vi "Update Controller State.vi"(8 "error in (no error)":errorcluster, 11 "ATM Controller in":refnum<class "ATM Controller.lvclass">) -> (0 "error out":errorcluster, 3 "ATM Controller out":refnum<class "ATM Controller.lvclass">)   [LabVIEW 2019, in "ATM Controller.lvlib" / "ATM Controller.lvclass"]
uses:
  ATM Controller.lvclass
  C:/Program Files (x86)/National Instruments/LabVIEW 2019/vi.lib/ActorFramework/Actor/Actor.lvclass
  <vilib>/ActorFramework/Actor/Actor.lvclass/Actor.ctl
  <vilib>/ActorFramework/Message Enqueuer/Message Enqueuer.lvclass/Message Enqueuer.ctl
  ATM Controller.lvclass/ATM Controller.ctl
  Sim Display Console Actor/ATM Controller/Transaction -Enum.ctl
  Sim Display Console Actor/ATM Controller/Message Name.ctl
  ATM Controller Messages/Set Message Msg/Set Message Msg.lvclass/Set Message Msg.ctl
  Sim User Console Actor/Sim User Console Actor Messages/Enable Transactions Msg/Enable Transactions Msg.lvclass/Enable Transactions Msg.ctl
  Sim User Console Actor/Sim User Console Actor Messages/Enable Keypad Msg/Enable Keypad Msg.lvclass/Enable Keypad Msg.ctl
  Sim User Console Actor/Sim User Console Actor Messages/Enable Card reader Msg/Enable Card reader Msg.lvclass/Enable Card reader Msg.ctl
  Sim Sensor Interface Actor/Sim Sensor Interface Actor Messages/Enable All Controls Msg/Enable All Controls Msg.lvclass/Enable All Controls Msg.ctl
  Sim Display Console Actor/Sim Display Console Actor Messages/Write Transaction Msg/Write Transaction Msg.lvclass/Write Transaction Msg.ctl
  Sim Display Console Actor/Sim Display Console Actor Messages/Write Card Read Msg/Write Card Read Msg.lvclass/Write Card Read Msg.ctl
  State -Enum.ctl
  ATM Controller Messages/Set Timer Msg/Set Timer Msg.lvclass/Set Timer Msg.ctl
  ATM Controller Messages/Set State Msg/Set State Msg.lvclass/Set State Msg.ctl
  Configuration Database/Configuration Database Messages/Read Record Msg/Read Record Msg.lvclass/Read Record Msg.ctl
  Sim User Console Actor/Sim User Console Actor Messages/Enable Terminate Session Msg/Enable Terminate Session Msg.lvclass/Enable Terminate Session Msg.ctl
  Sim User Console Actor/Sim User Console Actor Messages/Read New Transaction Msg/Read New Transaction Msg.lvclass/Read New Transaction Msg.ctl
  Configuration Database/Configuration Database/Record -Cluster.ctl
  Configuration Database/Configuration Database Messages/Write Record Msg/Write Record Msg.lvclass/Write Record Msg.ctl
  Sim Sensor Interface Actor/Sim Sensor Interface Actor Messages/Read Deposit Received Msg/Read Deposit Received Msg.lvclass/Read Deposit Received Msg.ctl
  Sim User Console Actor/Sim User Console Actor Messages/Enable New Transaction Msg/Enable New Transaction Msg.lvclass/Enable New Transaction Msg.ctl
  Sim Sensor Interface Actor/Sim Sensor Interface Actor Messages/Read Fund Dispensed Msg/Read Fund Dispensed Msg.lvclass/Read Fund Dispensed Msg.ctl
  <vilib>/ActorFramework/Message Enqueuer/Init from Existing Queue.vi
  <vilib>/ActorFramework/Message Enqueuer/Enqueue.vi
  ATM Controller Messages/Set Message Msg/Set Message Msg.lvclass
  C:/Program Files (x86)/National Instruments/LabVIEW 2019/vi.lib/ActorFramework/Message/Message.lvclass
  Sim Sensor Interface Actor/Sim Sensor Interface Actor Messages/Enable All Controls Msg/Enable All Controls Msg.lvclass
  Sim Display Console Actor/Sim Display Console Actor Messages/Write Transaction Msg/Write Transaction Msg.lvclass
  Sim Display Console Actor/Sim Display Console Actor Messages/Write Card Read Msg/Write Card Read Msg.lvclass
  Sim User Console Actor/Sim User Console Actor Messages/Enable Transactions Msg/Enable Transactions Msg.lvclass
  Sim User Console Actor/Sim User Console Actor Messages/Enable Keypad Msg/Enable Keypad Msg.lvclass
  Sim User Console Actor/Sim User Console Actor Messages/Enable Card reader Msg/Enable Card reader Msg.lvclass
  ATM Controller Messages/Set Timer Msg/Set Timer Msg.lvclass
  ATM Controller Messages/Set State Msg/Set State Msg.lvclass
  Configuration Database/Configuration Database Messages/Read Record Msg/Read Record Msg.lvclass
  Sim User Console Actor/Sim User Console Actor Messages/Enable Terminate Session Msg/Enable Terminate Session Msg.lvclass
  Sim User Console Actor/Sim User Console Actor Messages/Read New Transaction Msg/Read New Transaction Msg.lvclass
  Configuration Database/Configuration Database Messages/Write Record Msg/Write Record Msg.lvclass
  Sim Sensor Interface Actor/Sim Sensor Interface Actor Messages/Read Deposit Received Msg/Read Deposit Received Msg.lvclass
  Sim User Console Actor/Sim User Console Actor Messages/Enable New Transaction Msg/Enable New Transaction Msg.lvclass
  Sim Sensor Interface Actor/Sim Sensor Interface Actor Messages/Read Fund Dispensed Msg/Read Fund Dispensed Msg.lvclass
  <vilib>/ActorFramework/Message Priority Queue/Priority Enqueue.vi
  <vilib>/ActorFramework/Message Enqueuer/Message Enqueuer.lvclass
  <vilib>/ActorFramework/Actor/Actor.lvclass
  Sim Display Console Actor/ATM Controller/Sim Display Console Actor.lvclass
  Configuration Database/Configuration Database/Configuration Database.lvclass
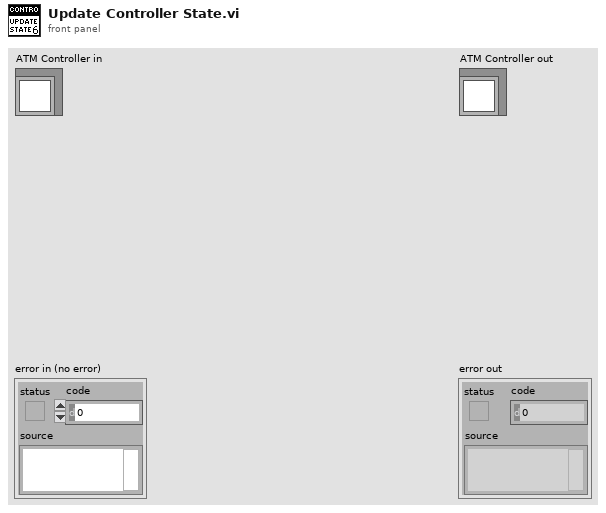
[diagram p1: front panel]
types:
  T1 = typedef "Sim Display Console Actor.lvlib/Sim Display Console Actor.lvclass/Message Name.ctl" = enum16{"Welcome", "Login", "Idle", "Invalid Login", "Terminate Session", "Deposit", "Withdrawal", "Fast Cash $50", "Withdrawal Complete", "Withdrawal Failed", "Balance Inquiry"}
  T2 = enum8{"Enabled", "Disabled", "Disabled and Grayed Out"}
  T3 = typedef "Sim Display Console Actor.lvlib/Sim Display Console Actor.lvclass/Transaction -Enum.ctl" = enum16{"", "Balance Inquiry", "Deposit", "Withdrawal", "Fast Cash $50", "New Transaction", "Terminate Session"}
  T4 = typedef "ATM Controller.lvlib/ATM Controller.lvclass/State -Enum.ctl" = enum16{"Initial", "Idle", "Login", "Balance Inquiry", "Deposit", "Withdrawal", "Fast Cash", "Terminate", "Inactivity Timeout"}
  T5 = typedef "Configuration Database.lvlib/Configuration Database.lvclass/Record -Cluster.ctl" = cluster{"First name":string, "Last Name":string, "Account Number":u16, "Balance":u32}
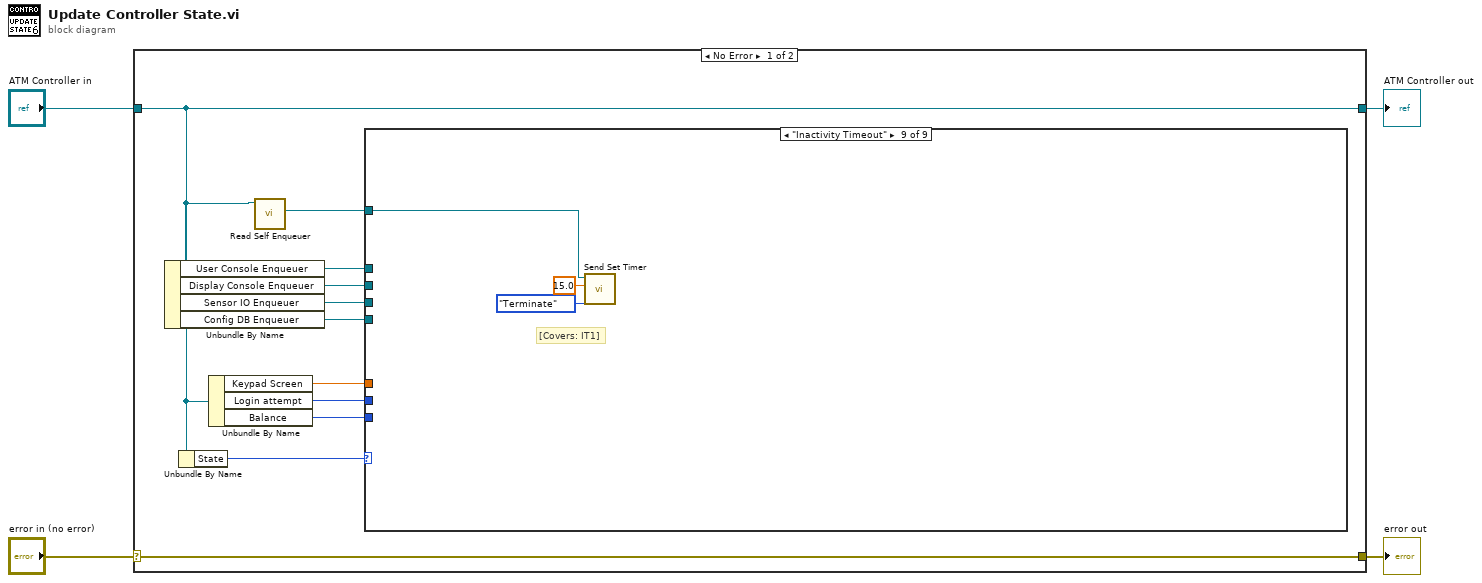
[diagram p0: block diagram]
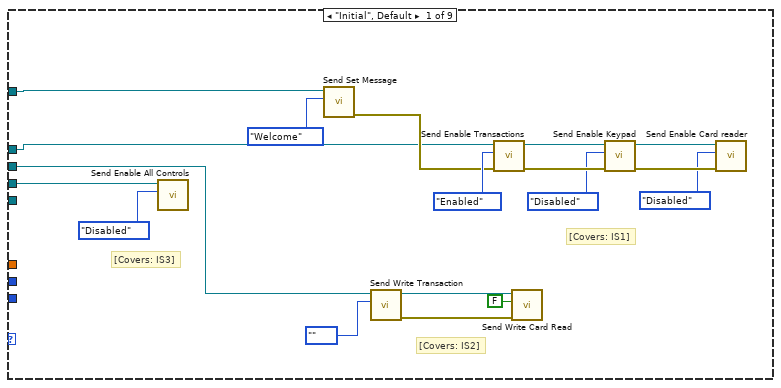
[diagram p2: hidden frame]
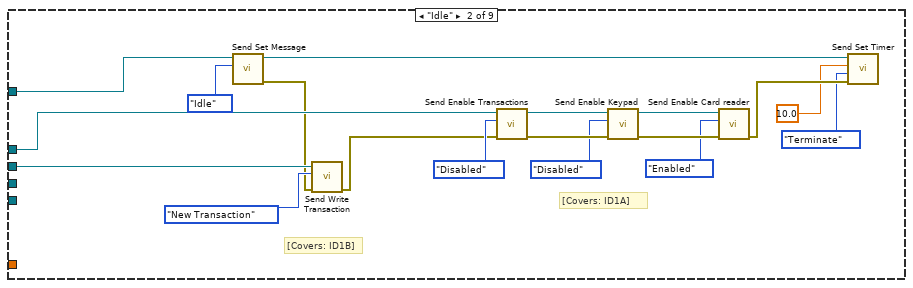
[diagram p3: hidden frame]
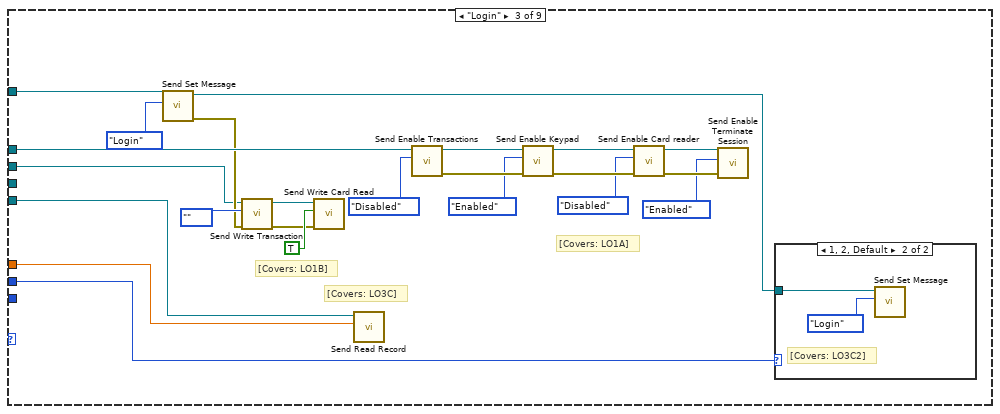
[diagram p4: hidden frame]
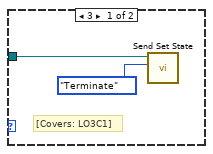
[diagram p5: hidden frame]
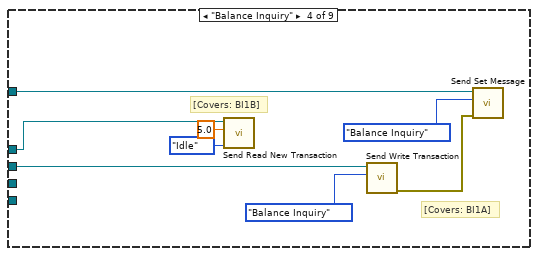
[diagram p6: hidden frame]
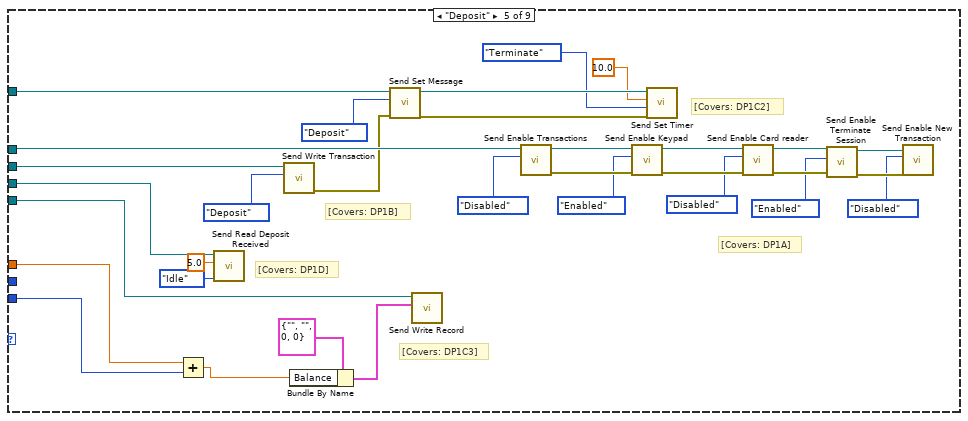
[diagram p7: hidden frame]
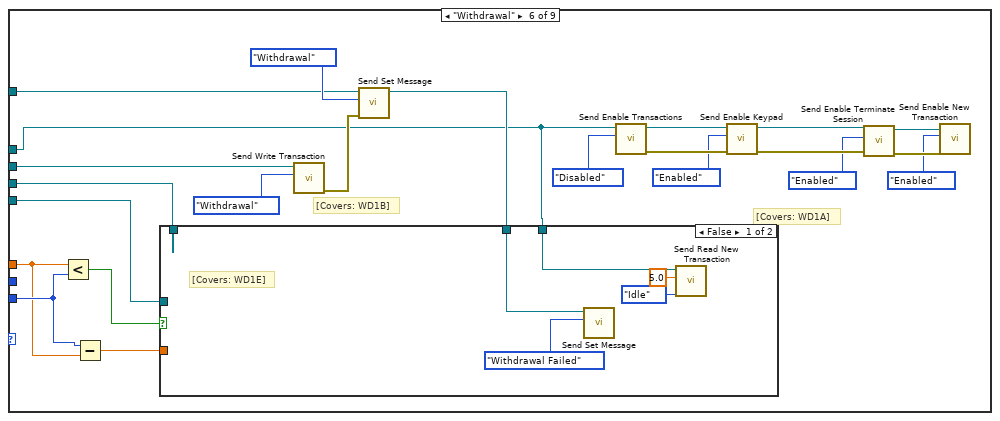
[diagram p8: hidden frame]
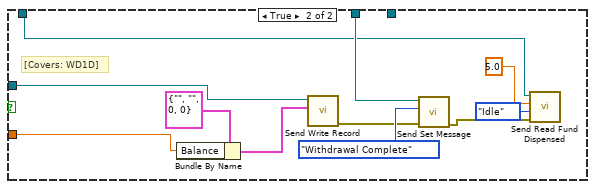
[diagram p9: hidden frame]
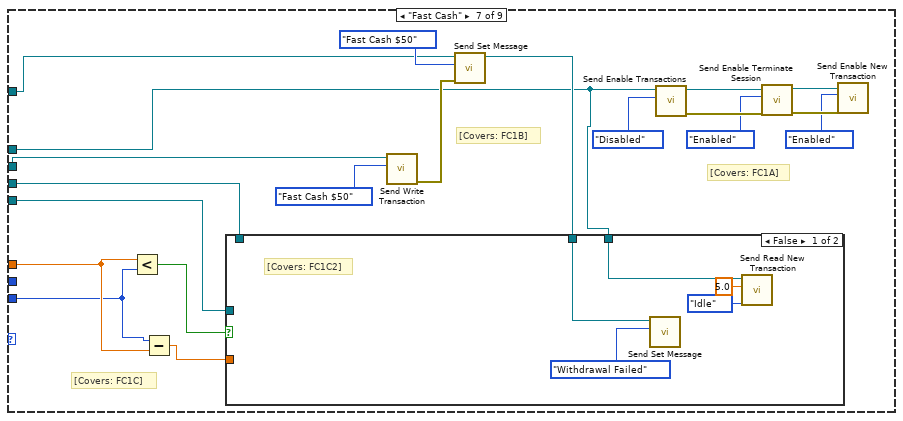
[diagram p10: hidden frame]
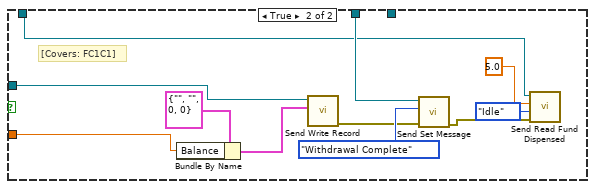
[diagram p11: hidden frame]
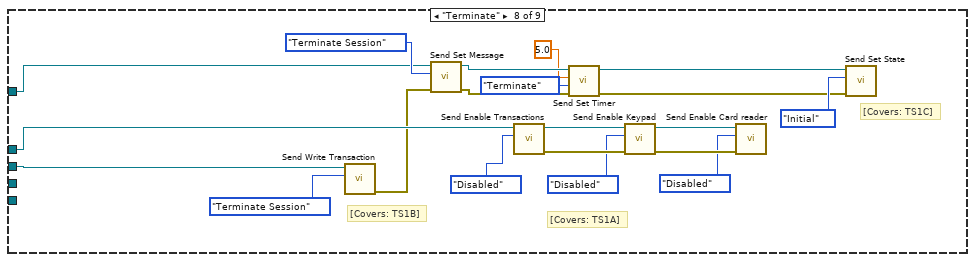
[diagram p12: hidden frame]
diagram:
  n1 = case shown="No Error" "error in (no error)" {
    selector: "error in (no error)" -> [w15 w218]
    tunnel: [w15 w218] -> w3
    tunnel: [w8 w217] -> w1
    tunnel: "ATM Controller in" -> [w8 w217]
    frame No Error {
      n2 = Unbundle By Name(w8) -> ("User Console Enqueuer"=w13:refnum<class "Message Enqueuer.lvclass">, "Display Console Enqueuer"=w12:refnum<class "Message Enqueuer.lvclass">, "Sensor IO Enqueuer"=w11:refnum<class "Message Enqueuer.lvclass">, "Config DB Enqueuer"=w10:refnum<class "Message Enqueuer.lvclass">)
      n3 = Unbundle By Name(w8) -> ("State"=w14:T4)
      n4 = Unbundle By Name(w8) -> ("Keypad Screen"=w7:dbl, "Login attempt"=w6:u8, "Balance"=w5:u32)
      n5 = call <vilib>:"Read Self Enqueuer.vi"("Actor"=w8) -> ("Self Enqueuer"=w9:refnum<class "Message Enqueuer.lvclass">)  [unwired: 10 in]
      n6 = case shown="\"Inactivity Timeout\"" w14 {
        tunnel: w13 -> [w17 w44 w67 w81 w109 w119 w158 w206 _]
        tunnel: w12 -> [w18 w40 w56 w86 w101 w127 w166 w202 _]
        tunnel: w11 -> [w22 _ _ _ w99 w120 w161 _ _]
        tunnel: w10 -> [_ _ w52 _ w98 w125 w160 _ _]
        tunnel: w9 -> [w16 w42 w60 w84 w100 w128 w168 w203 w214]
        tunnel: w7 -> [_ _ w53 _ w96 w123 w165 _ _]
        tunnel: w6 -> [_ _ w55 _ _ _ _ _ _]
        tunnel: w5 -> [_ _ _ _ w93 w124 w164 _ _]
        frame "Initial", Default {
          # "[Covers: IS3]"
          # "[Covers: IS2]"
          # "[Covers: IS1]"
          n7 = call "Send Enable All Controls.vi"("Disabled"=T2."Disabled", "Message Enqueuer"=w22) -> ()  [unwired: 8 in, 2 out]
          n8 = call "Send Set Message.vi"("Message Name"=Message_Name."Welcome", "Message Enqueuer"=w16) -> ("error out"=w19:errorcluster)  [unwired: 8 in, 1 out]
          n9 = call "Send Write Transaction.vi"("Transaction"=Transaction_-Enum."", "Message Enqueuer"=w18) -> ("error out"=w25:errorcluster, "Message Enqueuer out"=w26:refnum<class "Message Enqueuer.lvclass">)  [unwired: 8 in]
          n10 = call "Send Enable Transactions.vi"("error in (no error)"=w19, "Disabled"=T2."Enabled", "Message Enqueuer"=w17) -> ("error out"=w31:errorcluster, "Message Enqueuer out"=w33:refnum<class "Message Enqueuer.lvclass">)  [unwired: 7 in]
          n11 = call "Send Write Card Read.vi"("error in (no error)"=w25, "Card read"=FALSE, "Message Enqueuer"=w26) -> ()  [unwired: 7 in, 2 out]
          n12 = call "Send Enable Keypad.vi"("error in (no error)"=w31, "Disabled"=T2."Disabled", "Message Enqueuer"=w33) -> ("error out"=w30:errorcluster, "Message Enqueuer out"=w32:refnum<class "Message Enqueuer.lvclass">)  [unwired: 7 in]
          n13 = call "Send Enable Card reader.vi"("error in (no error)"=w30, "Disabled"=T2."Disabled", "Message Enqueuer"=w32) -> ()  [unwired: 7 in, 2 out]
        }
        frame "Idle" {
          # "[Covers: ID1B]"
          # "[Covers: ID1A]"
          n14 = call "Send Set Message.vi"("Message Name"=Message_Name."Idle", "Message Enqueuer"=w42) -> ("error out"=w39:errorcluster, "Message Enqueuer out"=w36:refnum<class "Message Enqueuer.lvclass">)  [unwired: 8 in]
          n15 = call "Send Write Transaction.vi"("error in (no error)"=w39, "Transaction"=Transaction_-Enum."New Transaction", "Message Enqueuer"=w40) -> ("error out"=w38:errorcluster)  [unwired: 7 in, 1 out]
          n16 = call "Send Enable Transactions.vi"("error in (no error)"=w38, "Disabled"=T2."Disabled", "Message Enqueuer"=w44) -> ("error out"=w49:errorcluster, "Message Enqueuer out"=w51:refnum<class "Message Enqueuer.lvclass">)  [unwired: 7 in]
          n17 = call "Send Enable Keypad.vi"("error in (no error)"=w49, "Disabled"=T2."Disabled", "Message Enqueuer"=w51) -> ("error out"=w48:errorcluster, "Message Enqueuer out"=w50:refnum<class "Message Enqueuer.lvclass">)  [unwired: 7 in]
          n18 = call "Send Enable Card reader.vi"("error in (no error)"=w48, "Disabled"=T2."Enabled", "Message Enqueuer"=w50) -> ("error out"=w37:errorcluster)  [unwired: 7 in, 1 out]
          n19 = call "Send Set Timer.vi"("error in (no error)"=w37, "State"=State_-Enum."Terminate", "Target time"=10.0, "Message Enqueuer"=w36) -> ()  [unwired: 6 in, 2 out]
        }
        frame "Login" {
          # "[Covers: LO3C]"
          # "[Covers: LO1B]"
          # "[Covers: LO1A]"
          n20 = call "Send Set Message.vi"("Message Name"=Message_Name."Login", "Message Enqueuer"=w60) -> ("error out"=w61:errorcluster, "Message Enqueuer out"=w54:refnum<class "Message Enqueuer.lvclass">)  [unwired: 8 in]
          n21 = call "Send Write Transaction.vi"("error in (no error)"=w61, "Transaction"=Transaction_-Enum."", "Message Enqueuer"=w56) -> ("error out"=w58:errorcluster, "Message Enqueuer out"=w57:refnum<class "Message Enqueuer.lvclass">)  [unwired: 7 in]
          n22 = call "Send Write Card Read.vi"("error in (no error)"=w58, "Card read"=TRUE, "Message Enqueuer"=w57) -> ()  [unwired: 7 in, 2 out]
          n23 = call "Send Read Record.vi"("Account Number"=w53, "Message Enqueuer"=w52) -> ()  [unwired: 8 in, 2 out]
          n24 = call "Send Enable Transactions.vi"("Disabled"=T2."Disabled", "Message Enqueuer"=w67) -> ("error out"=w72:errorcluster, "Message Enqueuer out"=w74:refnum<class "Message Enqueuer.lvclass">)  [unwired: 8 in]
          n25 = call "Send Enable Keypad.vi"("error in (no error)"=w72, "Disabled"=T2."Enabled", "Message Enqueuer"=w74) -> ("error out"=w71:errorcluster, "Message Enqueuer out"=w73:refnum<class "Message Enqueuer.lvclass">)  [unwired: 7 in]
          n26 = call "Send Enable Card reader.vi"("error in (no error)"=w71, "Disabled"=T2."Disabled", "Message Enqueuer"=w73) -> ("error out"=w66:errorcluster, "Message Enqueuer out"=w65:refnum<class "Message Enqueuer.lvclass">)  [unwired: 7 in]
          n27 = call "Send Enable Terminate Session.vi"("error in (no error)"=w66, "Disabled"=T2."Enabled", "Message Enqueuer"=w65) -> ()  [unwired: 7 in, 2 out]
          n28 = case shown="1, 2, Default" w55 {
            tunnel: w54 -> [w76 w78]
            frame 3 {
              # "[Covers: LO3C1]"
              n29 = call "Send Set State.vi"("State"=State_-Enum."Terminate", "Message Enqueuer"=w76) -> ()  [unwired: 8 in, 2 out]
            }
            frame 1, 2, Default {
              # "[Covers: LO3C2]"
              n30 = call "Send Set Message.vi"("Message Name"=Message_Name."Login", "Message Enqueuer"=w78) -> ()  [unwired: 8 in, 2 out]
            }
          }
        }
        frame "Balance Inquiry" {
          # "[Covers: BI1B]"
          # "[Covers: BI1A]"
          n31 = call "Send Read New Transaction.vi"("State"=State_-Enum."Idle", "Target time"=5.0, "Message Enqueuer"=w81) -> ()  [unwired: 7 in, 2 out]
          n32 = call "Send Write Transaction.vi"("Transaction"=Transaction_-Enum."Balance Inquiry", "Message Enqueuer"=w86) -> ("error out"=w82:errorcluster)  [unwired: 8 in, 1 out]
          n33 = call "Send Set Message.vi"("error in (no error)"=w82, "Message Name"=Message_Name."Balance Inquiry", "Message Enqueuer"=w84) -> ()  [unwired: 7 in, 2 out]
        }
        frame "Deposit" {
          # "[Covers: DP1C2]"
          # "[Covers: DP1D]"
          # "[Covers: DP1C3]"
          # "[Covers: DP1B]"
          # "[Covers: DP1A]"
          n34 = Add(x=w96, y=w93) -> (x+y=w95:dbl)
          n35 = call "Send Read Deposit Received.vi"("State"=State_-Enum."Idle", "Target time"=5.0, "Message Enqueuer"=w99) -> ()  [unwired: 7 in, 2 out]
          n36 = call "Send Write Transaction.vi"("Transaction"=Transaction_-Enum."Deposit", "Message Enqueuer"=w101) -> ("error out"=w102:errorcluster)  [unwired: 8 in, 1 out]
          n37 = Bundle By Name(cluster=T5 {"First name"="", "Last Name"="", "Account Number"=0, "Balance"=0} ("Record"), "Balance"=w95) -> (w94:T5)
          n38 = call "Send Set Message.vi"("error in (no error)"=w102, "Message Name"=Message_Name."Deposit", "Message Enqueuer"=w100) -> ("error out"=w90:errorcluster, "Message Enqueuer out"=w89:refnum<class "Message Enqueuer.lvclass">)  [unwired: 7 in]
          n39 = call "Send Write Record.vi"("Record"=w94, "Message Enqueuer"=w98) -> ()  [unwired: 8 in, 2 out]
          n40 = call "Send Enable Transactions.vi"("Disabled"=T2."Disabled", "Message Enqueuer"=w109) -> ("error out"=w116:errorcluster, "Message Enqueuer out"=w118:refnum<class "Message Enqueuer.lvclass">)  [unwired: 8 in]
          n41 = call "Send Enable Keypad.vi"("error in (no error)"=w116, "Disabled"=T2."Enabled", "Message Enqueuer"=w118) -> ("error out"=w115:errorcluster, "Message Enqueuer out"=w117:refnum<class "Message Enqueuer.lvclass">)  [unwired: 7 in]
          n42 = call "Send Set Timer.vi"("error in (no error)"=w90, "State"=State_-Enum."Terminate", "Target time"=10.0, "Message Enqueuer"=w89) -> ()  [unwired: 6 in, 2 out]
          n43 = call "Send Enable Card reader.vi"("error in (no error)"=w115, "Disabled"=T2."Disabled", "Message Enqueuer"=w117) -> ("error out"=w112:errorcluster, "Message Enqueuer out"=w111:refnum<class "Message Enqueuer.lvclass">)  [unwired: 7 in]
          n44 = call "Send Enable Terminate Session.vi"("error in (no error)"=w112, "Disabled"=T2."Enabled", "Message Enqueuer"=w111) -> ("error out"=w107:errorcluster, "Message Enqueuer out"=w106:refnum<class "Message Enqueuer.lvclass">)  [unwired: 7 in]
          n45 = call "Send Enable New Transaction.vi"("error in (no error)"=w107, "Disabled"=T2."Disabled", "Message Enqueuer"=w106) -> ()  [unwired: 7 in, 2 out]
        }
        frame "Withdrawal" {
          # "[Covers: WD1B]"
          # "[Covers: WD1A]"
          n46 = Less?(x=w123, y=w124) -> (x < y?=w126:bool)
          n47 = Subtract(x=w124, y=w123) -> (x-y=w122:dbl)
          n48 = call "Send Write Transaction.vi"("Transaction"=Transaction_-Enum."Withdrawal", "Message Enqueuer"=w127) -> ("error out"=w129:errorcluster)  [unwired: 8 in, 1 out]
          n49 = call "Send Set Message.vi"("error in (no error)"=w129, "Message Name"=Message_Name."Withdrawal", "Message Enqueuer"=w128) -> ("Message Enqueuer out"=w121:refnum<class "Message Enqueuer.lvclass">)  [unwired: 7 in, 1 out]
          n50 = case shown="False" w126 {
            tunnel: w125 -> [_ w155]
            tunnel: w122 -> [_ w154]
            tunnel: w121 -> [w146 w153]
            tunnel: w120 -> [_ w151]
            tunnel: w119 -> [w144 _]
            frame False {
              # "[Covers: WD1E]"
              n51 = call "Send Set Message.vi"("Message Name"=Message_Name."Withdrawal Failed", "Message Enqueuer"=w146) -> ()  [unwired: 8 in, 2 out]
              n52 = call "Send Read New Transaction.vi"("State"=State_-Enum."Idle", "Target time"=5.0, "Message Enqueuer"=w144) -> ()  [unwired: 7 in, 2 out]
            }
            frame True {
              # "[Covers: WD1D]"
              n53 = Bundle By Name(cluster=T5 {"First name"="", "Last Name"="", "Account Number"=0, "Balance"=0} ("Record"), "Balance"=w154) -> (w157:T5)
              n54 = call "Send Write Record.vi"("Record"=w157, "Message Enqueuer"=w155) -> ("error out"=w150:errorcluster)  [unwired: 8 in, 1 out]
              n55 = call "Send Set Message.vi"("error in (no error)"=w150, "Message Name"=Message_Name."Withdrawal Complete", "Message Enqueuer"=w153) -> ("error out"=w149:errorcluster)  [unwired: 7 in, 1 out]
              n56 = call "Send Read Fund Dispensed.vi"("error in (no error)"=w149, "State"=State_-Enum."Idle", "Target time"=5.0, "Message Enqueuer"=w151) -> ()  [unwired: 6 in, 2 out]
            }
          }
          n57 = call "Send Enable Transactions.vi"("Disabled"=T2."Disabled", "Message Enqueuer"=w119) -> ("error out"=w139:errorcluster, "Message Enqueuer out"=w141:refnum<class "Message Enqueuer.lvclass">)  [unwired: 8 in]
          n58 = call "Send Enable Keypad.vi"("error in (no error)"=w139, "Disabled"=T2."Enabled", "Message Enqueuer"=w141) -> ("error out"=w138:errorcluster, "Message Enqueuer out"=w140:refnum<class "Message Enqueuer.lvclass">)  [unwired: 7 in]
          n59 = call "Send Enable Terminate Session.vi"("error in (no error)"=w138, "Disabled"=T2."Enabled", "Message Enqueuer"=w140) -> ("error out"=w134:errorcluster, "Message Enqueuer out"=w133:refnum<class "Message Enqueuer.lvclass">)  [unwired: 7 in]
          n60 = call "Send Enable New Transaction.vi"("error in (no error)"=w134, "Disabled"=T2."Enabled", "Message Enqueuer"=w133) -> ()  [unwired: 7 in, 2 out]
        }
        frame "Fast Cash" {
          # "[Covers: FC1C]"
          # "[Covers: FC1B]"
          # "[Covers: FC1A]"
          n61 = Less?(x=w165, y=w164) -> (x < y?=w163:bool)
          n62 = Subtract(x=w164, y=w165) -> (x-y=w162:dbl)
          n63 = call "Send Write Transaction.vi"("Transaction"=Transaction_-Enum."Fast Cash $50", "Message Enqueuer"=w166) -> ("error out"=w167:errorcluster)  [unwired: 8 in, 1 out]
          n64 = call "Send Set Message.vi"("error in (no error)"=w167, "Message Name"=Message_Name."Fast Cash $50", "Message Enqueuer"=w168) -> ("Message Enqueuer out"=w159:refnum<class "Message Enqueuer.lvclass">)  [unwired: 7 in, 1 out]
          n65 = case shown="False" w163 {
            tunnel: w160 -> [_ w191]
            tunnel: w162 -> [_ w190]
            tunnel: w159 -> [w182 w189]
            tunnel: w161 -> [_ w187]
            tunnel: w158 -> [w180 _]
            frame False {
              # "[Covers: FC1C2]"
              n66 = call "Send Set Message.vi"("Message Name"=Message_Name."Withdrawal Failed", "Message Enqueuer"=w182) -> ()  [unwired: 8 in, 2 out]
              n67 = call "Send Read New Transaction.vi"("State"=State_-Enum."Idle", "Target time"=5.0, "Message Enqueuer"=w180) -> ()  [unwired: 7 in, 2 out]
            }
            frame True {
              # "[Covers: FC1C1]"
              n68 = Bundle By Name(cluster=T5 {"First name"="", "Last Name"="", "Account Number"=0, "Balance"=0} ("Record"), "Balance"=w190) -> (w193:T5)
              n69 = call "Send Write Record.vi"("Record"=w193, "Message Enqueuer"=w191) -> ("error out"=w186:errorcluster)  [unwired: 8 in, 1 out]
              n70 = call "Send Set Message.vi"("error in (no error)"=w186, "Message Name"=Message_Name."Withdrawal Complete", "Message Enqueuer"=w189) -> ("error out"=w185:errorcluster)  [unwired: 7 in, 1 out]
              n71 = call "Send Read Fund Dispensed.vi"("error in (no error)"=w185, "State"=State_-Enum."Idle", "Target time"=5.0, "Message Enqueuer"=w187) -> ()  [unwired: 6 in, 2 out]
            }
          }
          n72 = call "Send Enable Transactions.vi"("Disabled"=T2."Disabled", "Message Enqueuer"=w158) -> ("error out"=w176:errorcluster, "Message Enqueuer out"=w177:refnum<class "Message Enqueuer.lvclass">)  [unwired: 8 in]
          n73 = call "Send Enable Terminate Session.vi"("error in (no error)"=w176, "Disabled"=T2."Enabled", "Message Enqueuer"=w177) -> ("error out"=w173:errorcluster, "Message Enqueuer out"=w172:refnum<class "Message Enqueuer.lvclass">)  [unwired: 7 in]
          n74 = call "Send Enable New Transaction.vi"("error in (no error)"=w173, "Disabled"=T2."Enabled", "Message Enqueuer"=w172) -> ()  [unwired: 7 in, 2 out]
        }
        frame "Terminate" {
          # "[Covers: TS1C]"
          # "[Covers: TS1B]"
          # "[Covers: TS1A]"
          n75 = call "Send Write Transaction.vi"("Transaction"=Transaction_-Enum."Terminate Session", "Message Enqueuer"=w202) -> ("error out"=w201:errorcluster)  [unwired: 8 in, 1 out]
          n76 = call "Send Set Message.vi"("error in (no error)"=w201, "Message Name"=Message_Name."Terminate Session", "Message Enqueuer"=w203) -> ("error out"=w198:errorcluster, "Message Enqueuer out"=w199:refnum<class "Message Enqueuer.lvclass">)  [unwired: 7 in]
          n77 = call "Send Enable Transactions.vi"("Disabled"=T2."Disabled", "Message Enqueuer"=w206) -> ("error out"=w211:errorcluster, "Message Enqueuer out"=w213:refnum<class "Message Enqueuer.lvclass">)  [unwired: 8 in]
          n78 = call "Send Set Timer.vi"("error in (no error)"=w198, "State"=State_-Enum."Terminate", "Target time"=5.0, "Message Enqueuer"=w199) -> ("error out"=w197:errorcluster, "Message Enqueuer out"=w196:refnum<class "Message Enqueuer.lvclass">)  [unwired: 6 in]
          n79 = call "Send Enable Keypad.vi"("error in (no error)"=w211, "Disabled"=T2."Disabled", "Message Enqueuer"=w213) -> ("error out"=w210:errorcluster, "Message Enqueuer out"=w212:refnum<class "Message Enqueuer.lvclass">)  [unwired: 7 in]
          n80 = call "Send Enable Card reader.vi"("error in (no error)"=w210, "Disabled"=T2."Disabled", "Message Enqueuer"=w212) -> ()  [unwired: 7 in, 2 out]
          n81 = call "Send Set State.vi"("error in (no error)"=w197, "State"=State_-Enum."Initial", "Message Enqueuer"=w196) -> ()  [unwired: 7 in, 2 out]
        }
        frame "Inactivity Timeout" {
          # "[Covers: IT1]"
          n82 = call "Send Set Timer.vi"("State"=State_-Enum."Terminate", "Target time"=15.0, "Message Enqueuer"=w214) -> ()  [unwired: 7 in, 2 out]
        }
      }
    }
    frame Error {
    }
  }
  "error out" <- w3
  "ATM Controller out" <- w1
